vi "Command Turn to Heading Speed Cap.vi"(7 "Startup":bool, 9 "Timeout":dbl=15.0, 10 "Max Speed":dbl, 11 "Heading":dbl=-90.0) -> (2 "Right Wheel Velocity":dbl=680.96, 3 "Left Wheel Velocity":dbl=-680.96, 4 "Reint":bool, 6 "Completed":bool)   [LabVIEW 2017]
uses:
  Command Execution State.ctl
  Utility VIs/Refnum Names.vi
  Drive/Drive Globals.vi
  <vilib>/Rock Robotics/WPI/ThirdParty/Phoenix-LabVIEW/Pigeon IMU/CTRE_PigeonIMU_GetRawGyro.vi
panel:
  in  "Increment":dbl=1.2
  out "Out Speed":cluster{dbl, dbl}(graph)
  out "Turn Speed":cluster{"Command ":dbl, dbl, dbl}(graph)
  out "Using Lower?":bool=TRUE
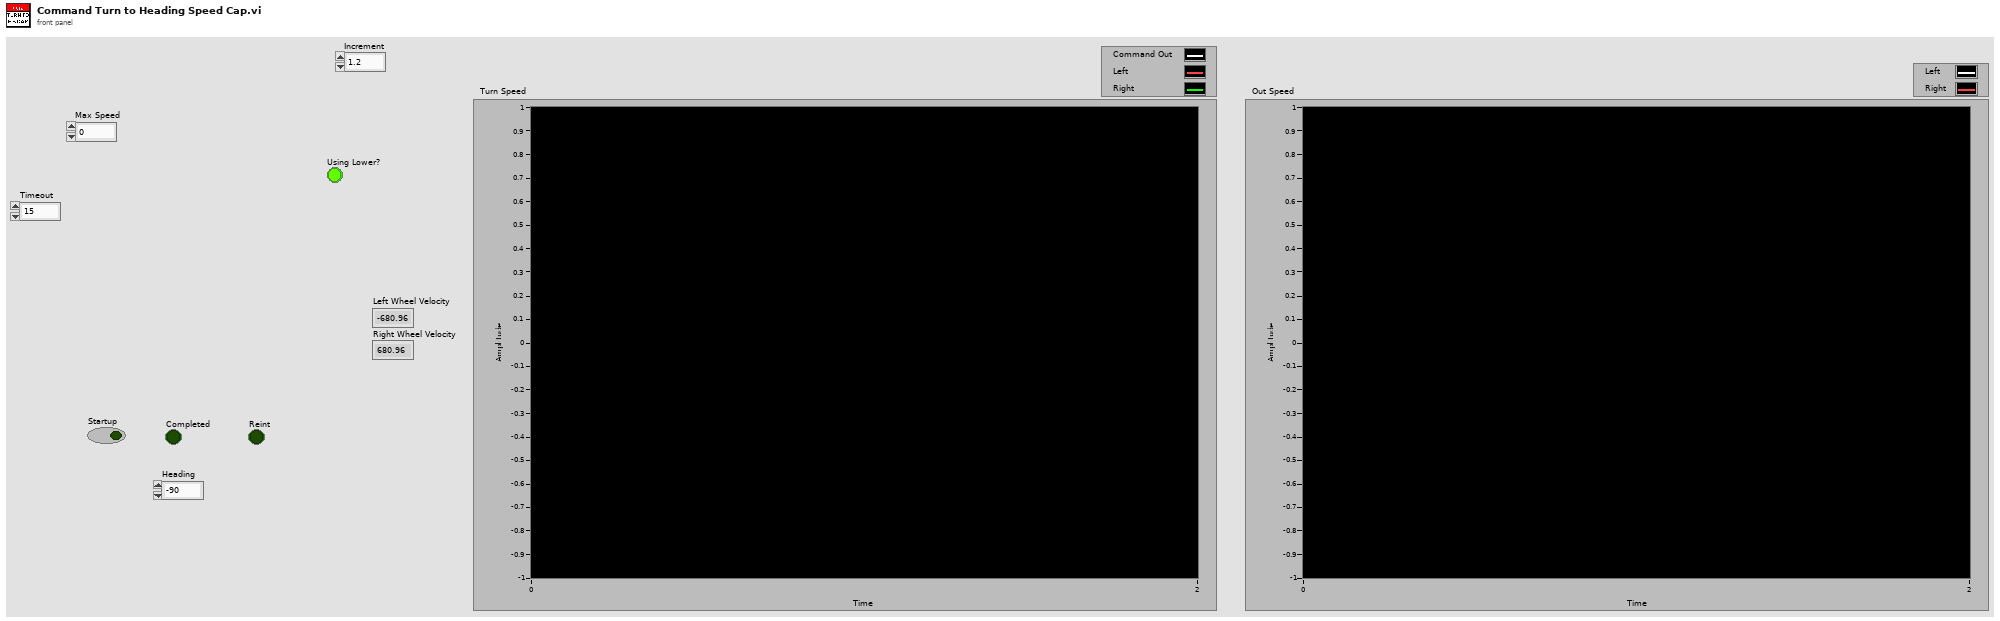
[diagram p1: front panel]
types:
  T1 = typedef "Command Execution State.ctl" = enum16{"Initialize", "Execute", "Finish"}
  T2 = typedef "CTRE_PigeonIMU_DeviceRef.ctl" = cluster{"DeviceStatus":errorcluster, "Device Number":u8, "Type":T3, "Device ID":u32, "Handle":u64, "UsageFrame":u32, "Library Path":path}
  T3 = typedef "CTRE_PigeonIMU_ConnectionType.ctl" = u32
  T4 = cluster{"X":dbl, "Y":dbl, "Z":dbl, "Magnitude":dbl}
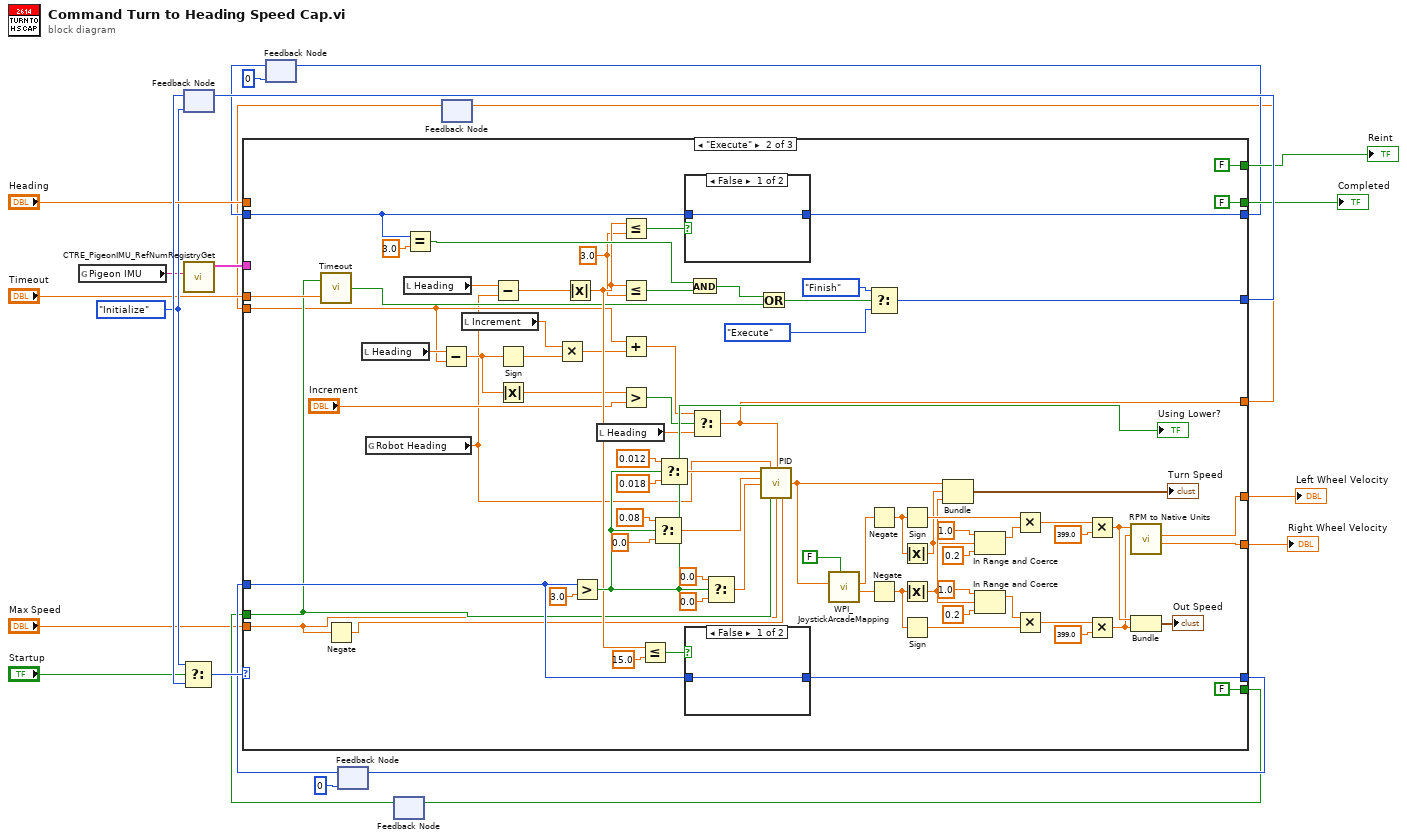
[diagram p0: block diagram]
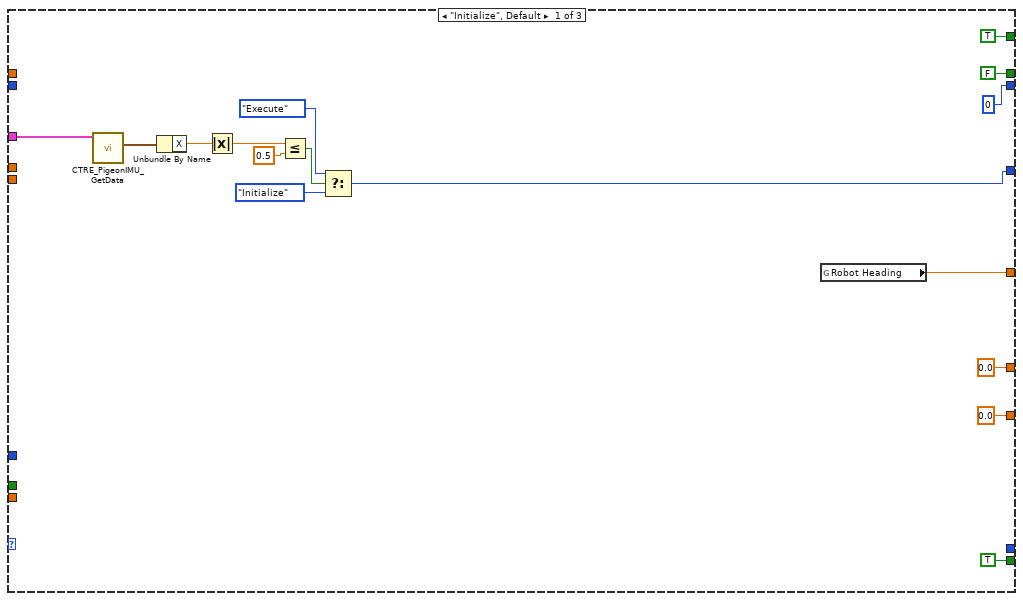
[diagram p2: hidden frame]
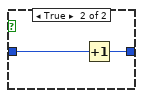
[diagram p3: hidden frame]
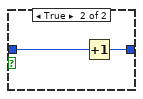
[diagram p4: hidden frame]
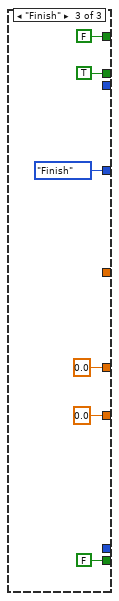
[diagram p5: hidden frame]
diagram:
  w20 = Command_Execution_State."Initialize" ("Play State")
  n1 = global read "Refnum Names.vi" "Pigeon IMU"() -> (w11:string)
  n2 = feedback #1(w20) -> (w22:T1)
  n3 = Select(t=w20, s="Startup", f=w22) -> (s? t:f=w24:T1)
  n4 = call <vilib>:"CTRE_PigeonIMU_RefNumRegistryGet.vi"("refnum name"=w11) -> ("PigeonIMUDevRef"=w10:T2)  [unwired: 9 in, 1 out]
  n5 = feedback #2(0) -> (w13:i32)
  n6 = feedback #3(0 ("y")) -> (w9:i32)
  n7 = feedback #4() -> (w4:bool)  [unwired: 1 in]
  n8 = feedback #5() -> (w1:dbl)  [unwired: 1 in]
  n9 = case shown="\"Execute\"" w24 {
    tunnel: [w32 w114 Command_Execution_State."Finish" ("Play State")] -> w23
    tunnel: "Heading" -> [_ _ _]
    tunnel: [FALSE FALSE TRUE] -> w19
    tunnel: [TRUE FALSE FALSE] -> w17
    tunnel: [0.0 w79 0.0] -> w16
    tunnel: [0.0 w78 0.0] -> w15
    tunnel: w13 -> [_ w106 _]
    tunnel: [0 w107 _] -> w12
    tunnel: w10 -> [w34 _ _]
    tunnel: w9 -> [_ w95 _]
    tunnel: [_ w96 _] -> w8
    tunnel: "Timeout" -> [_ w83 _]
    tunnel: [TRUE FALSE FALSE] -> w5
    tunnel: w4 -> [_ w67 _]
    tunnel: "Max Speed" -> [_ w65 _]
    tunnel: [w25 w49 _] -> w2
    tunnel: w1 -> [_ w48 _]
    frame "Initialize", Default {
      n10 = call-poly <vilib>:"CTRE_PigeonIMU_GetData.vi"("PigeonIMUDevRef"=w34) -> ("Gyro DPS"=w35:T4)  [unwired: 8 in, 2 out]
      n11 = Unbundle By Name(w35) -> ("X"=w31:dbl)
      n12 = Absolute Value(x=w31) -> (abs(x)=w29:dbl)
      n13 = Less Or Equal?(x=w29, y=0.5) -> (x <= y?=w28:bool)
      n14 = Select(t=Command_Execution_State."Execute" ("Play State"), s=w28, f=Command_Execution_State."Initialize") -> (s? t:f=w32:T1)
      n15 = global read "Drive Globals.vi" "Robot Heading"() -> (w25:dbl)
    }
    frame "Execute" {
      w76 = 3.0 ("t")
      n16 = call "Timeout.vi"("Timeout"=w83, "Initialize"=w67) -> ("Timed Out?"=w81:bool)
      n17 = Negate(x=w65) -> (-x=w66:dbl)
      n18 = local read "Heading"() -> (w55:dbl)
      n19 = global read "Drive Globals.vi" "Robot Heading"() -> (w41:dbl)
      n20 = local read "Heading"() -> (w42:dbl)
      n21 = Equal?(x=w106, y=3.0 ("t")) -> (x = y?=w101:bool)
      n22 = Subtract(x=w55, y=w48) -> (x-y=w45:dbl)
      n23 = local read "Increment"() -> (w44:dbl)
      n24 = Subtract(x=w42, y=w41) -> (x-y=w43:dbl)
      n25 = Sign(1:w45) -> (0:w46:dbl)
      n26 = Absolute Value(x=w45) -> (abs(x)=w52:dbl)
      n27 = Multiply(x=w44, y=w46) -> (x*y=w47:dbl)
      n28 = Absolute Value(x=w43) -> (abs(x)=w98:dbl)
      n29 = Greater?(x=w95, y=3.0 ("t")) -> (0:w102:bool)
      "Using Lower?" <- w102
      n30 = local read "Heading"() -> (w50:dbl)
      n31 = Less Or Equal?(x=w98, y=w76) -> (x <= y?=w112:bool)
      n32 = Less Or Equal?(x=w98, y=w76) -> (x <= y?=w99:bool)
      n33 = Add(x=w48, y=w47) -> (x+y=w51:dbl)
      n34 = Greater?(x=w52, y="Increment") -> (0:w53:bool)
      n35 = Less Or Equal?(x=w98, y=15.0 ("t")) -> (x <= y?=w97:bool)
      n36 = Select(t=0.08, s=w102, f=0.0 ("t")) -> (s? t:f=w103:dbl)
      n37 = Select(t=0.012, s=w102, f=0.018 ("t")) -> (s? t:f=w105:dbl)
      n38 = case shown="False" w112 {
        tunnel: w106 -> [w121 w123]
        tunnel: [w121 w122] -> w107
        frame False {
        }
        frame True {
          n39 = Increment(x=w123) -> (x+1=w122:i32)
        }
      }
      n40 = case shown="False" w97 {
        tunnel: w95 -> [w118 w120]
        tunnel: [w118 w119] -> w96
        frame False {
        }
        frame True {
          n41 = Increment(x=w120) -> (x+1=w119:i32)
        }
      }
      n42 = And(x=w101, y=w99) -> (x .and. y?=w100:bool)
      n43 = Select(t=w51, s=w53, f=w50) -> (s? t:f=w49:dbl)
      n44 = Select(t=0.0, s=w102, f=0.0 ("t")) -> (s? t:f=w104:dbl)
      n45 = Or(x=w100, y=w81) -> (x .or. y?=w82:bool)
      n46 = call "PID.vi"("Kp"=w105, "Process Variable"=w41, "Goal"=w49, "Ki"=w103, "Kd"=w104, "Reinit"=w67, "Max Ouput"=w65, "Min Output"=w66) -> ("Command"=w59:dbl)  [unwired: 5 in, 2 out]
      n47 = call <vilib>:"WPI_JoystickArcadeMapping.vi"("Square Inputs"=FALSE, "X axis value"=w59) -> ("Right Motor Value"=w110:dbl, "Left Motor Value"=w111:dbl)  [unwired: 8 in]
      n48 = Select(t=Command_Execution_State."Finish" ("Play State"), s=w82, f=Command_Execution_State."Execute") -> (s? t:f=w114:T1)
      n49 = Negate(x=w111) -> (-x=w87:dbl)
      n50 = Negate(x=w110) -> (-x=w86:dbl)
      n51 = Sign(1:w87) -> (0:w94:dbl)
      n52 = Absolute Value(x=w87) -> (abs(x)=w57:dbl)
      n53 = Absolute Value(x=w86) -> (abs(x)=w58:dbl)
      n54 = Sign(1:w86) -> (0:w91:dbl)
      n55 = Bundle("Command"=w59, w57, w58) -> (→"Turn Speed":cluster{"Command ":dbl, dbl, dbl})  [unwired: 1 in]
      n56 = In Range and Coerce(upper limit=1.0, x=w57, lower limit=0.2) -> (coerced(x)=w93:dbl)  [unwired: 1 out]
      n57 = In Range and Coerce(upper limit=1.0, x=w58, lower limit=0.2) -> (coerced(x)=w92:dbl)  [unwired: 1 out]
      n58 = Multiply(x=w94, y=w93) -> (x*y=w84:dbl)
      n59 = Multiply(x=w92, y=w91) -> (x*y=w85:dbl)
      n60 = Multiply(x=w84, y=399.0) -> (x*y=w63:dbl)
      n61 = Multiply(x=w85, y=399.0) -> (x*y=w62:dbl)
      n62 = call "RPM to Native Units.vi"("Right RPM"=w62, "Left RPM"=w63) -> ("Right Out"=w78:dbl, "Left Out"=w79:dbl)  [unwired: 6 in, 1 out]
      n63 = Bundle(w63, w62) -> (→"Out Speed":cluster{dbl, dbl})  [unwired: 1 in]
    }
    frame "Finish" {
    }
  }
  "Completed" <- w19
  "Reint" <- w17
  "Left Wheel Velocity" <- w16
  "Right Wheel Velocity" <- w15
  n64 = feedback-in #1(w23) -> ()
  n65 = feedback-in #2(w12) -> ()
  n66 = feedback-in #3(w8) -> ()
  n67 = feedback-in #4(w5) -> ()
  n68 = feedback-in #5(w2) -> ()
